vi "convert 1D image array to 2D image - U8 input.vi"(8 "Height":i64(slide)=1200 min=0 max=1200 step=4 scale=0.0..1200.0, 9 "Width":i64(slide)=1920 min=0 max=1920 step=4 scale=0.0..1920.0, 11 "Image Data Array":u8[](array[numeric])) -> (3 "Intensity Graph":u8[][](graph))   [LabVIEW 2020]
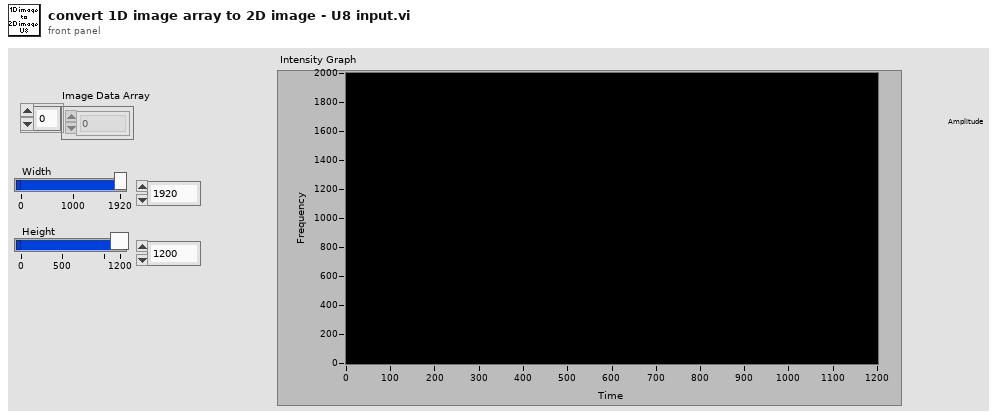
[diagram p1: front panel]
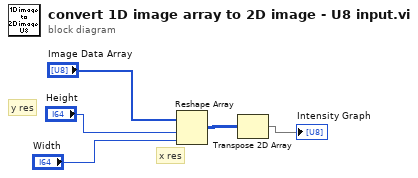
[diagram p0: block diagram]
diagram:
  # "x res"
  # "y res"
  n1 = Reshape Array("Image Data Array", "Height", "Width") -> (w5:u8[][])
  n2 = Transpose 2D Array(2D array=w5) -> (transposed array=→"Intensity Graph":u8[][])
